vi "configuration to node.vi"(8 "error in":errorcluster, 10 "configuration":refnum<class "NISE_CEF_serializable configuration.lvclass">, 11 "hierarchy repo in":refnum<class "NISE_CEF_HierarchyRepo.lvclass">) -> (0 "error out":errorcluster, 2 "node":refnum<class "NISE_CEF_serializable node.lvclass">, 3 "hierarchy repo out":refnum<class "NISE_CEF_HierarchyRepo.lvclass">)   [LabVIEW 2013, in "NISE_CEF_HierarchyRepo.lvclass"]
uses:
  NISE_CEF_HierarchyRepo.lvclass
  serializable configuration/NISE_CEF_serializable configuration.lvclass
  serializable node/NISE_CEF_serializable node.lvclass
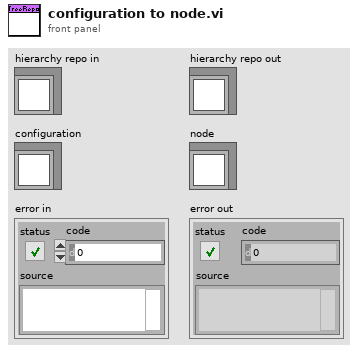
[diagram p1: front panel]
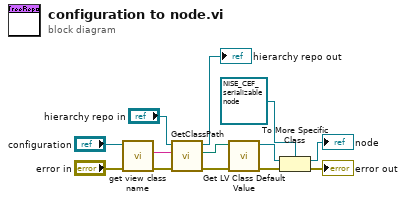
[diagram p0: block diagram]
diagram:
  n1 = call "get view class name.vi"("error in"="error in", "configuration in"="configuration") -> ("error out"=w9:errorcluster, "view class"=w8:string)  [unwired: 7 in, 1 out]
  n2 = call-dynamic "GetClassPath.vi"("error in"=w9, "class name"=w8, "Repository in"="hierarchy repo in") -> ("error out"=w6:errorcluster, "class path"=w7:path, "Repository out"=→"hierarchy repo out":refnum<class "NISE_CEF_HierarchyRepo.lvclass">)  [unwired: 6 in]
  n3 = call <vilib>:"Get LV Class Default Value.vi"("error in (no error)"=w6, "class path"=w7) -> ("error out"=w5:errorcluster, "object"=w4:refnum<class>)  [unwired: 8 in]
  n4 = To More Specific Class(target class=refnum<class "NISE_CEF_serializable node.lvclass"> refnum ("node"), reference=w4, error in=w5) -> (specific class reference=→"node":refnum<class "NISE_CEF_serializable node.lvclass">, error out=→"error out":errorcluster)
